vi "Steam Set S&THx.vi"() -> ()   [LabVIEW 2017]
panel:
  out "Steam Set":dbl
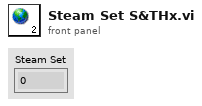
[diagram p1: front panel]
diagram:
